vi "移位寄存器（累乘累加）.vi"() -> ()   [LabVIEW 2017]
panel:
  out "累乘":i32
  out "累加":i32
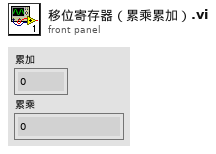
[diagram p1: front panel]
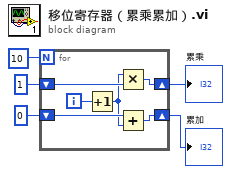
[diagram p0: block diagram]
diagram:
  n1 = for {
    N: 10 -> [_]
    shift-right: [w10] -> w3
    shift-left: 0 -> [w11]
    shift-right: [w7] -> w1
    shift-left: 1 -> [w8]
    i -> [w9]
    n2 = Increment(x=w9) -> (x+1=w6:i32)
    n3 = Multiply(x=w6, y=w8) -> (x*y=w7:i32)
    n4 = Add(x=w11, y=w6) -> (x+y=w10:i32)
  }
  "累加" <- w3
  "累乘" <- w1
